vi "linear_forward.vi"(2 "b":dbl[][](array[numeric]), 3 "W":dbl[][](array[numeric]), 4 "A":dbl[][](array[numeric])) -> (0 "cache":cluster{"A":dbl[][], "W":dbl[][], "b":dbl[][]}, 1 "Z":dbl[][](array[numeric]))   [LabVIEW 2020]
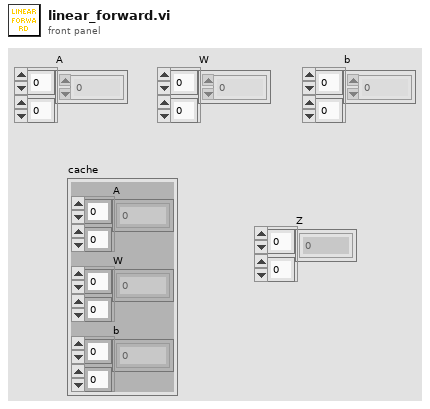
[diagram p1: front panel]
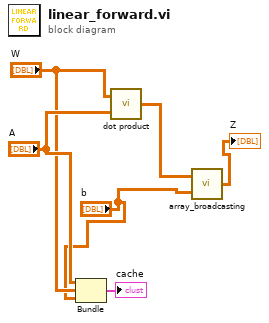
[diagram p0: block diagram]
diagram:
  n1 = Bundle("A"="A", "W"="W", "b"="b") -> (→"cache":cluster{"A":dbl[][], "W":dbl[][], "b":dbl[][]})  [unwired: 1 in]
  n2 = call "dot product.vi"("y"="A", "x"="W") -> ("dot(x,y)"=w2:dbl[][])
  n3 = call "array_broadcasting.vi"("broad_array"="b", "Array"=w2) -> ("sum()"=→"Z":dbl[][])
